vi "binningsize.vi"(2 "CCD Binning":dbl, 3 "Software Binning":T1={"Software\nBinning?"=FALSE, "Software Bin Size"=1}) -> (0 "Software Bin Size":i32, 1 "Binning Value":dbl)   [LabVIEW 2013]
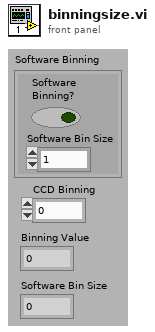
[diagram p1: front panel]
types:
  T1 = cluster{"Software\nBinning?":bool, "Software Bin Size":i32}
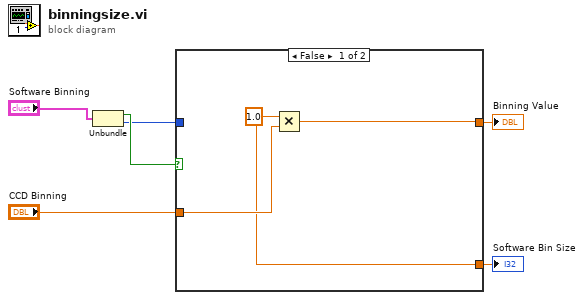
[diagram p0: block diagram]
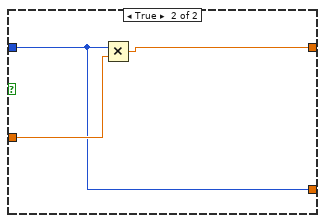
[diagram p2: hidden frame]
diagram:
  n1 = Unbundle("Software Binning") -> ("Software\nBinning?"=w5:bool, "Software Bin Size"=w4:i32)
  n2 = case shown="False" w5 {
    tunnel: w4 -> [_ w10]
    tunnel: [w8 w11] -> w2
    tunnel: "CCD Binning" -> [w9 w12]
    tunnel: [w7 w10] -> w1
    frame False {
      w7 = 1.0 ("x")
      n3 = Multiply(x=w7, y=w9) -> (x*y=w8:dbl)
    }
    frame True {
      n4 = Multiply(x=w10, y=w12) -> (x*y=w11:dbl)
    }
  }
  "Binning Value" <- w2
  "Software Bin Size" <- w1
